vi "Read Temp.vi"(8 "error in (no error)":errorcluster, 11 "Sim Laser Driver in":refnum<class "Sim Laser Driver.lvclass">) -> (0 "error out":errorcluster, 2 "Temp":dbl, 3 "Sim Laser Driver out":refnum<class "Sim Laser Driver.lvclass">)   [LabVIEW 2022 SP3, in "Sim Laser Driver.lvclass"]
uses:
  Sim Laser Driver.lvclass
  Accessors/Read Current Temp.vi
  Accessors/Read Warming.vi
  Accessors/Write Current Temp.vi
  Sim Laser Driver.lvclass/Sim Laser Driver.ctl
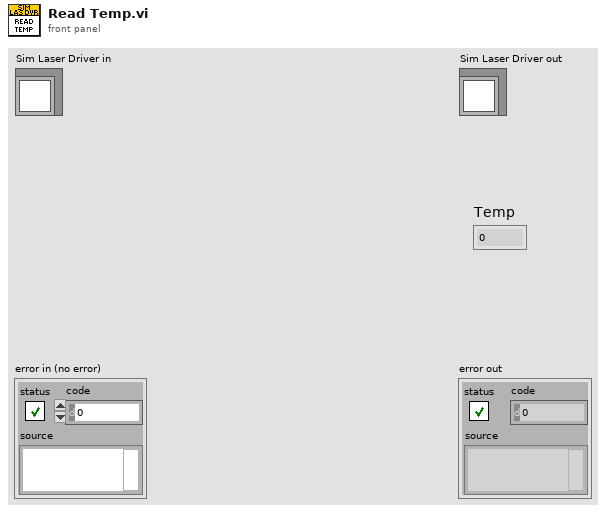
[diagram p1: front panel]
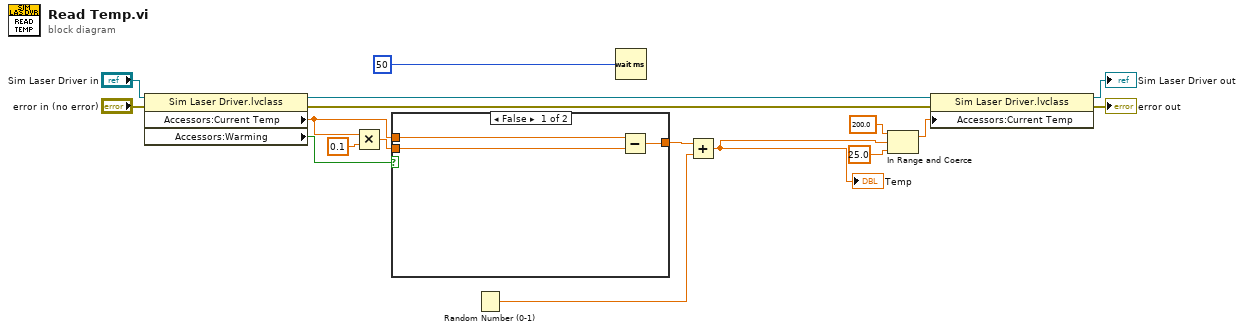
[diagram p0: block diagram]
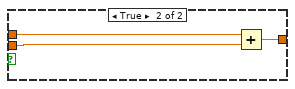
[diagram p2: hidden frame]
diagram:
  n1 = property class="Sim Laser Driver.lvclass"(reference="Sim Laser Driver in", error in="error in (no error)") -> (reference out=w16:refnum<class "Sim Laser Driver.lvclass">, error out=w5:errorcluster, "Accessors:Current Temp"=w13:dbl, "Accessors:Warming"=w8:bool)
  n2 = Multiply(x=w13, y=0.1) -> (x*y=w14:dbl)
  n3 = case shown="False" w8 {
    tunnel: w14 -> [w20 w23]
    tunnel: w13 -> [w19 w22]
    tunnel: [w18 w21] -> w11
    frame False {
      n4 = Subtract(x=w19, y=w20) -> (x-y=w18:dbl)
    }
    frame True {
      n5 = Add(x=w22, y=w23) -> (x+y=w21:dbl)
    }
  }
  n6 = Random Number (0-1)() -> (number: 0 to 1=w1:dbl)
  n7 = Wait (ms)(milliseconds to wait=u32 50) -> ()  [unwired: 1 out]
  n8 = Add(x=w11, y=w1) -> (x+y=w2:dbl)
  "Temp" <- w2
  n9 = In Range and Coerce(upper limit=200.0, x=w2, lower limit=25.0) -> (coerced(x)=w9:dbl)  [unwired: 1 out]
  n10 = property class="Sim Laser Driver.lvclass"(reference=w16, error in=w5, "Accessors:Current Temp"=w9) -> (reference out=→"Sim Laser Driver out":refnum<class "Sim Laser Driver.lvclass">, error out=→"error out":errorcluster)
